vi "Connect Channels (Single).vi"(8 "error in (no error)":errorcluster, 9 "channel 2":string, 10 "channel 1":string, 11 "session in":T1) -> (0 "error out":errorcluster, 3 "session out":T1)   [LabVIEW 2020, in "SLSC Switch.lvlib"]
doc: "Creates a path between <B>channel 1</B> and <B>channel 2</B>. NI-SLSC Switch calculates and uses the shortest path between the two channels. Refer to Setting Source and Configuration Channels for information about channel usage types."
uses:
  <vilib>/SLSC_Switch/SLSC Switch.lvlib
  nislscsl.dll
  <vilib>/userdefined/High Color/SLSC_Switch/nislscslSession.ctl
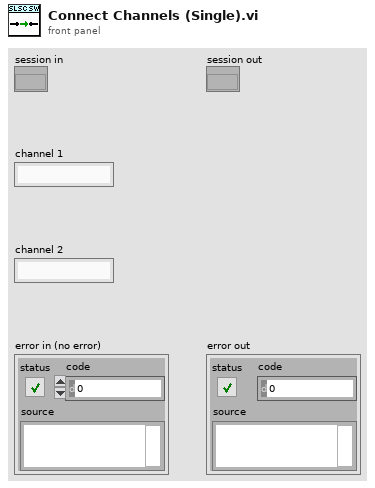
[diagram p1: front panel]
types:
  T1 = typedef "nislscslSession.ctl" = refnum<k20>
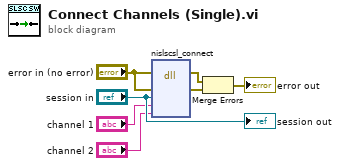
[diagram p0: block diagram]
diagram:
  n1 = dll-call lib="nislscsl.*" fn="nislscsl_connect"(error in="error in (no error)", "errorCluster"="error in (no error)", "sessionHandle"="session in", "channel1"="channel 1", "channel2"="channel 2") -> (error out=w7:errorcluster, "errorCluster"=w6:errorcluster)  [unwired: 6 in, 1 out]
  n2 = Merge Errors(w7, w6) -> (→"error out":errorcluster)
  "session out" <- "session in"
